vi "FindArrayCtlRefs.vi"(8 "error in (no error)":errorcluster, 10 "CLT Ref Array":refnum<vi>[](array[refnum]), 11 "CTL Name Array":string[](array[string])) -> (0 "error out":errorcluster, 2 "Cluster CTL Array":refnum<vi>[](array[refnum]), 3 "Cluster CTL Name Array":string[](array[string]))   [LabVIEW 2020, in "CtlReferences.lvlib" / "CtlReferences.lvclass"]
doc: "Get the refs of the CTLS in a Cluster.\nThis VI will also get the CTLS of any clusters inside the cluster... etc."
uses:
  CtlReferences.lvclass
  TypeDefs/ClassID_Enum.ctl
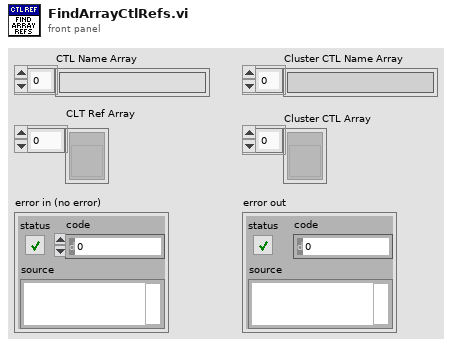
[diagram p1: front panel]
types:
  T1 = typedef "CtlReferences.lvlib/CtlReferences.lvclass/ClassID_Enum.ctl" = enum32{"0 <undefined>", "1 <undefined>", "2 <undefined>", "Generic", "Decoration", "Text", "Control", "ColorBox", "Boolean", "RefNum", "Variant", "Path", "ListBox", "Table", "Array", "Picture", "ActiveXContainer", "Numeric", "Digital", "NamedNumeric", "ColorRamp", "Slide", "GraphOrChart", "WaveformChart", "WaveformGraph", "IntensityChart", "IntensityGraph", "String", "IOName", "ComboBox", "Cluster", "Panel", "Knob", "NumWithScale", "Ring", "Enum", "GObject", "Plot", "Cursor", "NumericText", "Scale", "ColorScale", "GraphScale", "ColorGraphScale", "TypedRefNum", "OldKnobScale", "MCListbox", "MeasureData", "BVTag", "DAQName", "VISAName", "IVIName", "SlideScale", "TabControl", "Page", "TabArrayTabControl", "ConPane"}
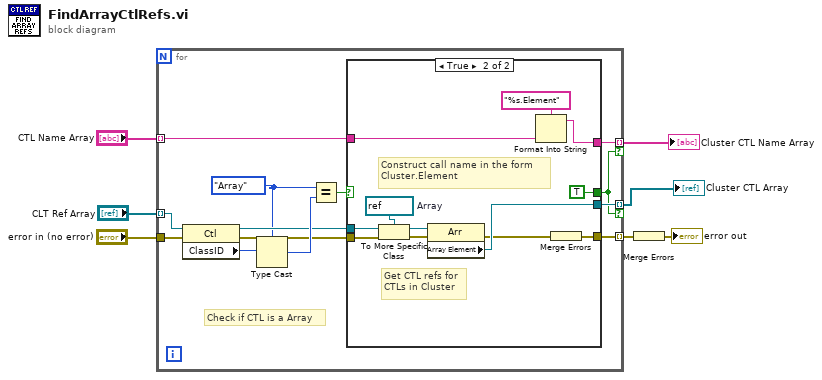
[diagram p0: block diagram]
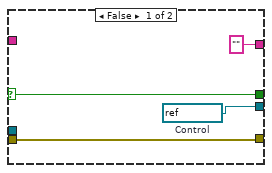
[diagram p2: hidden frame]
diagram:
  n1 = for {
    tunnel: "error in (no error)" -> [w14]
    tunnel: "CTL Name Array" -> [w19] mode=indexing
    tunnel: [w18] -> w1 mode=indexing if=w15
    tunnel: [w17] -> w7 mode=indexing
    tunnel: [w16] -> w2 mode=indexing if=w15
    tunnel: "CLT Ref Array" -> [w13] mode=indexing
    w8 = ClassID_Enum."Array" ("ClassID Name")
    # "Check if CTL is a Array"
    n2 = property class="Ctl"(reference=w13, error in=w14) -> (reference out=w10:refnum<vi>, error out=w9:errorcluster, "ClassID"=w12:u32)
    n3 = Type Cast(type=w8, x=w12) -> (*(type *) &x=w11:T1)
    n4 = Equal?(x=w8, y=w11) -> (x = y?=w20:bool)
    n5 = case shown="True" w20 {
      selector: w20 -> [w23 _]
      tunnel: w9 -> [w24 w36]
      tunnel: w10 -> [_ w26]
      tunnel: w19 -> [_ w30]
      tunnel: [w21 w32] -> w18
      tunnel: [w24 w29] -> w17
      tunnel: ["" w28] -> w16
      tunnel: [w23 TRUE] -> w15
      frame False {
        w21 = refnum<vi> refnum  # Control
      }
      frame True {
        w35 = refnum<vi> refnum  # Array
        # "Construct call name in the form\nCluster.Element"
        # "Get CTL refs for\nCTLs in Cluster"
        n6 = To More Specific Class(target class=w35, reference=w26, error in=w36) -> (specific class reference=w34:refnum<vi>, error out=w33:errorcluster)
        n7 = property class="Arr"(reference=w34, error in=w33) -> (error out=w31:errorcluster, "Array Element"=w32:refnum<vi>)  [unwired: 1 out]
        n8 = Format Into String(format string="%s.Element", w30) -> (resulting string=w28:string)  [unwired: 2 in, 1 out]
        n9 = Merge Errors(w31) -> (w29:errorcluster)
      }
    }
  }
  "Cluster CTL Name Array" <- w2
  "Cluster CTL Array" <- w1
  n10 = Merge Errors(w7) -> (→"error out":errorcluster)
